vi "TestInitializeLocalLogSingleAbstractSink_NoLogInstantiated.vi"(8 "error in (no error)":errorcluster, 11 "TestCase in":refnum<class "TestMalleableInterface.lvclass">) -> (0 "error out":errorcluster, 3 "TestCase out":refnum<class "TestMalleableInterface.lvclass">)   [LabVIEW 2017, in "TestMalleableInterface.lvclass"]
uses:
  TestMalleableInterface.lvclass
  Source/Composed Log/Log Sink/Log Sink.lvclass
  Source/Composed Log/LoggerReference/LoggerReference.lvclass/LoggerReference.ctl
  8d299841-f253-422a-a7a1-59edf70c310f.vi
  Source/Composed Log/LoggerReference/Return Aggregate Queues.vi
  Source/Composed Log/LoggerReference/Add Aggregate Log.vi
  8d299841-f253-422a-a7a1-59edf70c310f.vi/5d8b6823-3e6c-4102-8691-68f09e549259.vi
  Source/Composed Log/LoggerReference/Send Add Sink.vi
  Source/Composed Log/Application Logger/Launch Worker Loop.vi
  Source/Composed Log/LoggerReference/Initialize Logger Instance.vi
  Source/Composed Log/LoggerReference/LoggerReference.lvclass
  Source/Composed Log/IErrorFormat/IErrorFormat.lvclass
  <vilib>/addons/_JKI Toolkits/VI Tester/TestCase.llb/TestCase.lvclass
  C:/Program Files (x86)/National Instruments/LabVIEW 2017/vi.lib/addons/_JKI Toolkits/VI Tester/TestCase.llb/TestCase.lvclass
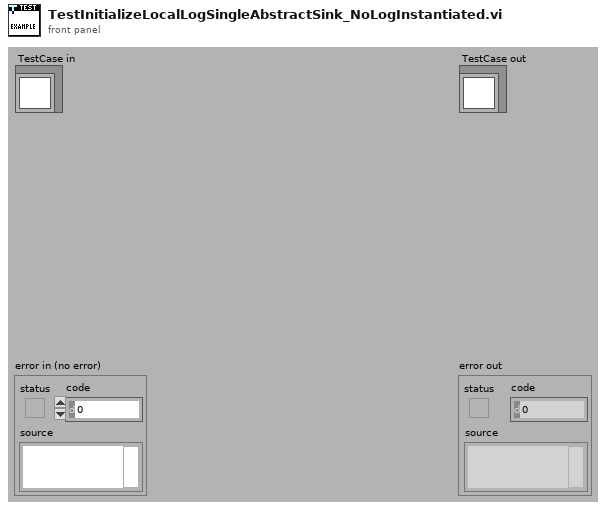
[diagram p1: front panel]
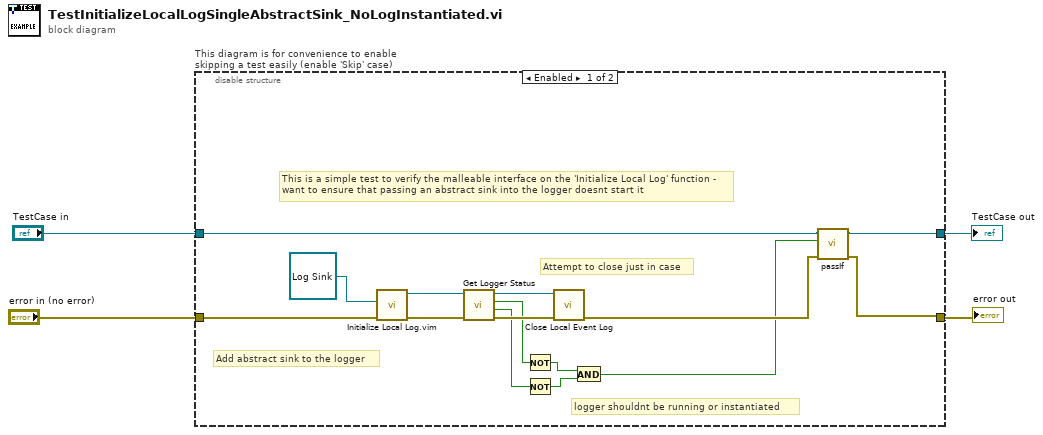
[diagram p0: block diagram]
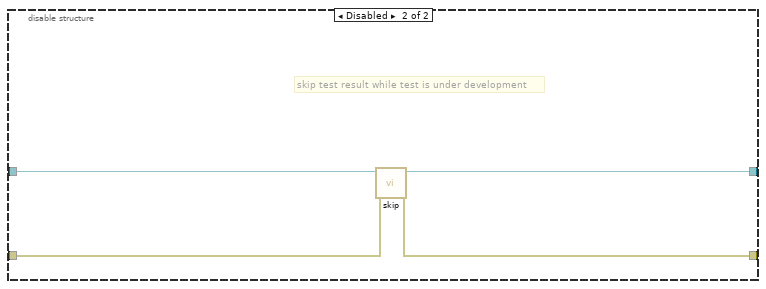
[diagram p2: hidden frame]
diagram:
  n1 = disable-structure "This diagram is for convenience to enable skipping a test easily (enable 'Skip' case)" shown="Enabled" {
    disable-tunnel: "TestCase in" -> [w16 w23]
    disable-tunnel: [w15 w21] -> w1
    disable-tunnel: [w14 w22] -> w3
    disable-tunnel: "error in (no error)" -> [w19 w20]
    frame Enabled {
      # "logger shouldnt be running or instantiated"
      # "Attempt to close just in case"
      # "This is a simple test to verify the malleable interface on the 'Initialize Local Log' function - want to ensure that passing an abstract sink into the logger doesnt start it"
      # "Add abstract sink to the logger"
      n2 = call "Initialize Local Log.vim"("error in (no error)"=w19, "Startup Sink(s)"=refnum<class "Log Sink.lvclass"> refnum) -> ("error out"=w12:errorcluster, "Log Instance Reference"=w13:refnum<class "LoggerReference.lvclass">)  [unwired: 7 in, 1 out]
      n3 = call "Get Logger Status.vi"("error in (no error)"=w12, "LoggerReference in"=w13) -> ("error out"=w11:errorcluster, "Logger Running?"=w8:bool, "Logger Instantiated?"=w9:bool, "LoggerReference out"=w10:refnum<class "LoggerReference.lvclass">)  [unwired: 6 in]
      n4 = Not(x=w9) -> (.not. x?=w7:bool)
      n5 = Not(x=w8) -> (.not. x?=w6:bool)
      n6 = call "Close Local Event Log.vi"("error in (no error)"=w11, "Log Instance"=w10) -> ("error out"=w17:errorcluster)  [unwired: 9 in]
      n7 = And(x=w7, y=w6) -> (x .and. y?=w5:bool)
      n8 = call-dynamic "passIf.vi"("error in (no error)"=w17, "pass"=w5, "TestCase in"=w16) -> ("error out"=w14:errorcluster, "TestCase out"=w15:refnum<class "TestMalleableInterface.lvclass">)  [unwired: 7 in]
    }
    frame Disabled {
      # "skip test result while test is under development"
      n9 = call <vilib>:"skip.vi"("error in (no error)"=w20, "TestCase in"=w23) -> ("error out"=w22:errorcluster, "TestCase out"=w21:refnum<class "TestMalleableInterface.lvclass">)  [unwired: 8 in]
    }
  }
  "error out" <- w3
  "TestCase out" <- w1
